vi "GetID.vi"(8 "Fehler (Eingang, kein Fehler)":errorcluster caption="Error_In", 11 "OXYGEN Ref In":refnum<visa-resource-name>) -> (0 "Fehler (Ausgang)":errorcluster caption="Error_Out", 1 "Raw communication data":T1, 2 "Device Identification":string, 3 "OXYGEN Ref Out":refnum<visa-resource-name>)   [LabVIEW 2018, in "OXYGEN.lvlib"]
doc: "Query the ID string of the instrument."
uses:
  OXYGEN.lvlib
  TypeDefs/Cluster_RawCommData.ctl
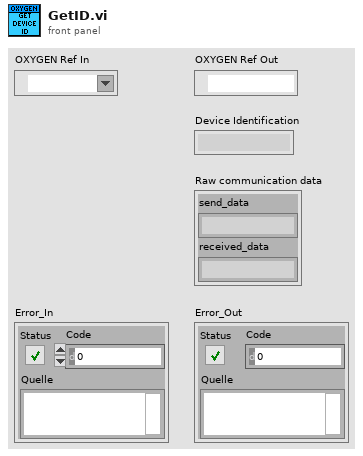
[diagram p1: front panel]
types:
  T1 = typedef "OXYGEN.lvlib/Cluster_RawCommData.ctl" = cluster{"send_data":string, "received_data":string}
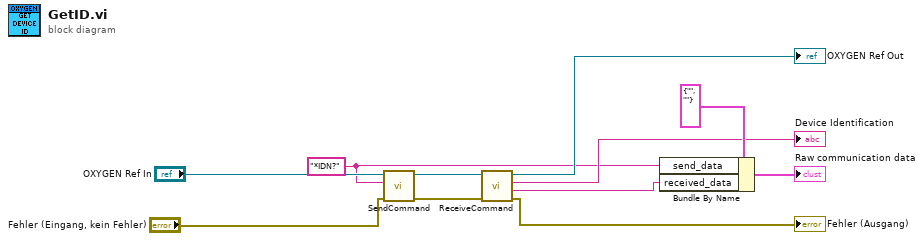
[diagram p0: block diagram]
diagram:
  w2 = "*IDN?" ("Schreibpuffer")
  n1 = call "SendCommand.vi"("error in (no error)"="Fehler (Eingang, kein Fehler)", "String to Send"=w2, "OXY_SCPI Reseource In"="OXYGEN Ref In") -> ("error out"=w6:errorcluster, "OXY_SCPI Reseource Out"=w7:refnum<visa-resource-name>)  [unwired: 7 in]
  n2 = call "ReceiveCommand.vi"("error in (no error)"=w6, "OXY_SCPI Reseource In"=w7) -> ("error out"=→"Fehler (Ausgang)":errorcluster, "received Data with Header"=w1:string, "received Data"=→"Device Identification":string, "OXY_SCPI Reseource Out"=→"OXYGEN Ref Out":refnum<visa-resource-name>)  [unwired: 6 in]
  n3 = Bundle By Name(cluster=T1 {"send_data"="", "received_data"=""} ("communication_data"), "send_data"=w2, "received_data"=w1) -> (→"Raw communication data":T1)
